vi "Write CData.vi"(8 "error in (no error)":errorcluster, 10 "CData":T1, 11 "CData in":refnum<class "CData.lvclass">) -> (0 "error out":errorcluster, 3 "CData out":refnum<class "CData.lvclass">)   [LabVIEW 2014, in "CData.lvclass"]
uses:
  CData.lvclass
  Controls/CData Core Control.ctl
  Controls/File Data.ctl
  Libraries/Contact Data/Contact.ctl
  Libraries/Contact Data/Position.ctl
  Libraries/Contact Data/Controls.ctl
  Libraries/Contact Data/DestinationCluster.ctl
  Libraries/Contact Data/DesinationControls.ctl
  CData.lvclass/CData.ctl
  Libraries/Contact Data/Contact Data.lvlib
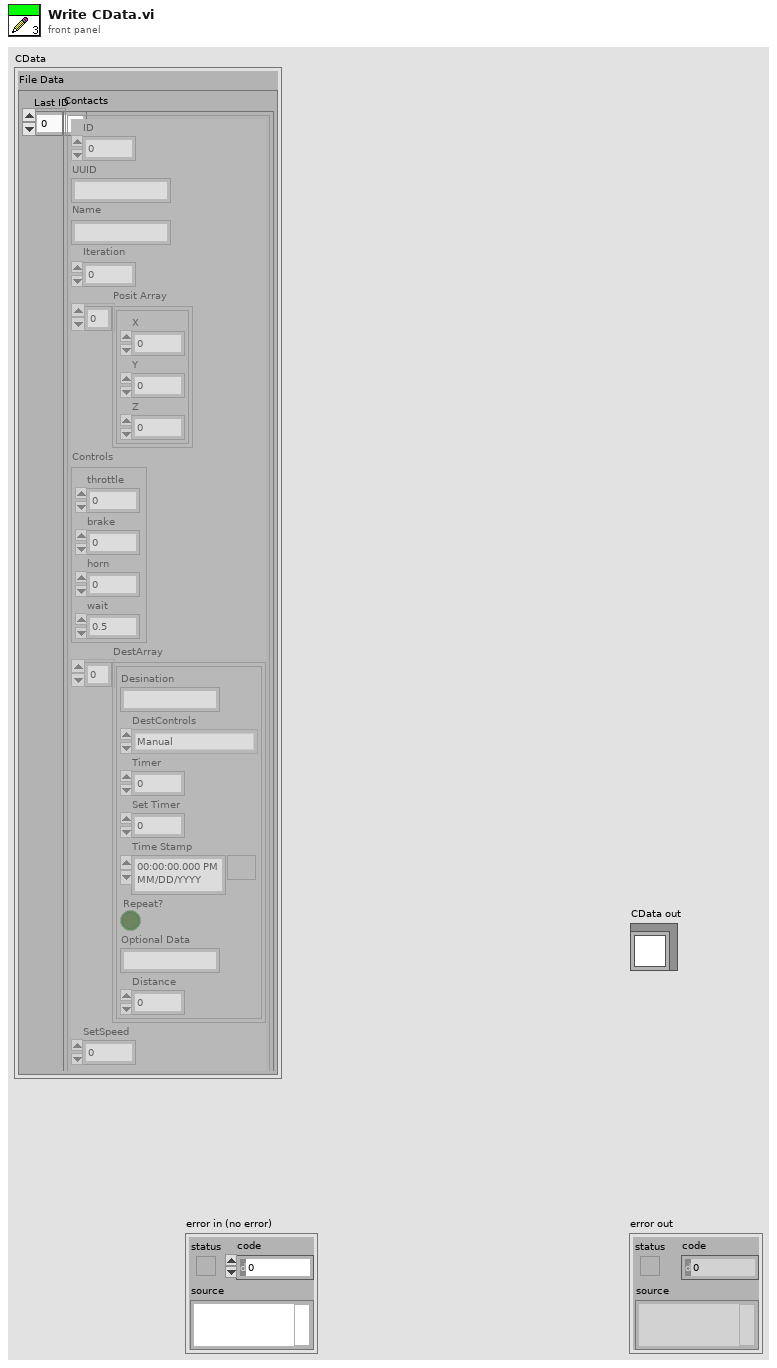
[diagram p1: front panel]
types:
  T1 = typedef "CData Core Control.ctl" = cluster{"File Data":T2}
  T2 = typedef "File Data.ctl" = cluster{"Last ID":u32, "Contacts":T3[]}
  T3 = typedef "Contact Data.lvlib/Contact.ctl" = cluster{"ID":u32, "UUID":string, "Name":string, "Iteration":i32, "Posit Array":T4[], "Controls":T5, "DestArray":T6[], "SetSpeed":dbl, "Speed":dbl}
  T4 = typedef "Contact Data.lvlib/Position.ctl" = cluster{"X":dbl, "Y":dbl, "Z":dbl}
  T5 = typedef "Contact Data.lvlib/Controls.ctl" = cluster{"throttle":dbl, "brake":dbl, "horn":dbl, "wait":dbl}
  T6 = typedef "Contact Data.lvlib/DestinationCluster.ctl" = cluster{"Desination":string, "DestControls":T7, "Timer":u32, "Set Timer":u32, "Time Stamp":timestamp, "Repeat?":bool, "Optional Data":string, "Distance":dbl}
  T7 = typedef "Contact Data.lvlib/DesinationControls.ctl" = enum16{"Tracker", "Manual", "Stop", "Station DateTime", "Station Timer", "Maintain"}
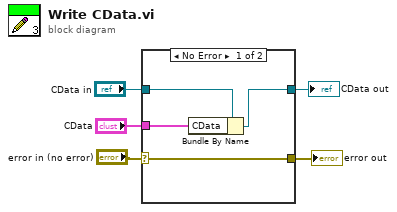
[diagram p0: block diagram]
diagram:
  n1 = case shown="No Error" "error in (no error)" {
    selector: "error in (no error)" -> [w9 w11]
    tunnel: [w9 w11] -> w4
    tunnel: [w7 w10] -> w2
    tunnel: "CData in" -> [w8 w10]
    tunnel: "CData" -> [w6 _]
    frame No Error {
      n2 = Bundle By Name(cluster=w8, "CData"=w6) -> (w7:refnum<class "CData.lvclass">)
    }
    frame Error {
    }
  }
  "error out" <- w4
  "CData out" <- w2
